vi "Constants.vi"() -> ()   [LabVIEW 2016, in "LIN Frame Protection Addon Shared.lvlib"]
doc: "Use this Global VI to access the GUIDs assigned to the page resources of the Custom Device."
uses:
  LIN Frame Protection Addon Shared.lvlib
panel:
  in  "Tab Control":enum32{"GUIDS", "Constants", "Properties"}(tab)
  in  "Rolling Counter Channel":string="7762d13c-0e79-4a98-8860-3f1fdd9b969e"
  in  "Protection Valid Channel":string="9276a97d-3f8a-408d-abe9-bee8bcaeaa49"
  in  "Protection Channel":string="6cc69156-b54d-4826-9e4e-4b8a23c5091b"
  in  "Monitor Page":string="46c0c29d-91f6-4a25-a156-b8ef24eac378"
  in  "Generate Page":string="f13b48ba-08da-41b2-b56f-dc3afba5b864"
  in  "Frame Configuration Page":string="080faed8-00b0-4df2-aec4-78e1bf3caf32"
  in  "LIN Frame Protection Addon":string="ce747db1-c753-4820-92b9-411d84571b92"
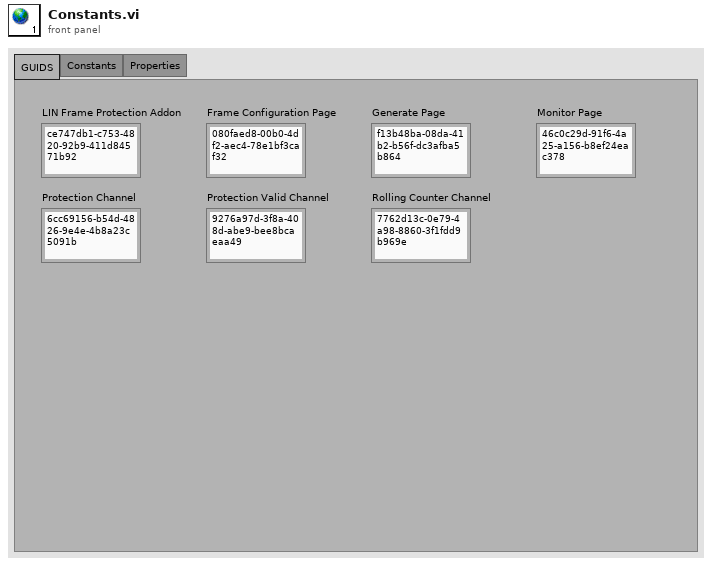
[diagram p1: front panel]
diagram:
